vi "Call.vi"(7 "Actor in":refnum<class "Actor.lvclass">, 8 "Error in":errorcluster, 10 "Msg":refnum<class "Msg.lvclass">) -> (0 "Error out":errorcluster, 2 "Msg Output":refnum<class "Msg Output.lvclass">, 5 "Actor out":refnum<class "Actor.lvclass">)   [LabVIEW 2020, in "jettl.lvlib"]
uses:
  jettl.lvlib
  Actor/Actor.lvclass
  Msg Output/Msg Output.lvclass
  Msg/Msg.lvclass
  Default Implementation.vi
  Attributes/Attributes.lvclass
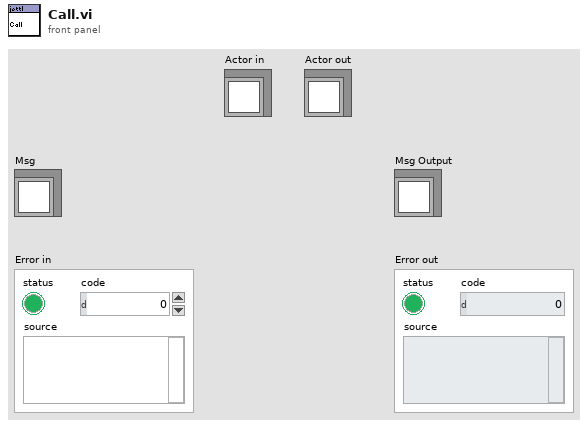
[diagram p1: front panel]
types:
  T1 = typedef "jettl.lvlib/Msgs.ctl" = set{refnum<class "Msg.lvclass">}
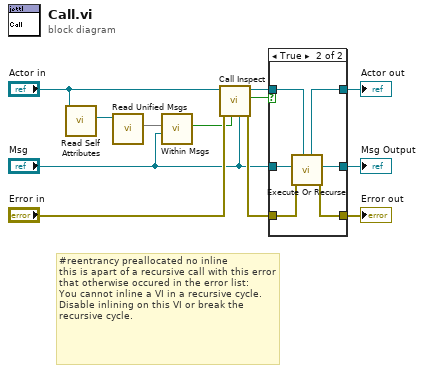
[diagram p0: block diagram]
diagram:
  # "#reentrancy preallocated no inline\nthis is apart of a recursive call with this error that otherwise occured in the error list:\nYou cannot inline a VI in a recursive cycle. Disable inlining on this VI or break the recursive cycle."
  n1 = call-dynamic "Read Self Attributes.vi"("Actor in"="Actor in") -> ("Self Attributes"=w12:refnum<class "Attributes.lvclass">)  [unwired: 10 in]
  n2 = call-dynamic "Read Unified Msgs.vi"("Attributes in"=w12) -> ("Unified Msgs"=w11:T1)  [unwired: 10 in]
  n3 = call "Within Msgs.vi"("Msg"="Msg", "Msgs"=w11) -> ("Within Msgs"=w1:bool)  [unwired: 9 in]
  n4 = call-dynamic "Call Inspect.vi"("Msg"="Msg", "Within Unified Msgs"=w1, "Error in"="Error in", "Actor in"="Actor in") -> ("Error out"=w3:errorcluster, "Proceed"=w5:bool, "Actor out"=w7:refnum<class "Actor.lvclass">)  [unwired: 5 in]
  n5 = case shown="True" w5 {
    tunnel: w7 -> [w14 w20]
    tunnel: [w14 w19] -> w9
    tunnel: "Msg" -> [_ w17]
    tunnel: [w13 w18] -> w8
    tunnel: [_ w16] -> w6
    tunnel: w3 -> [w13 w15]
    frame False {
    }
    frame True {
      n6 = call "Execute Or Recurse.vi"("Actor in"=w20, "Error in"=w15, "Msg"=w17) -> ("Error out"=w18:errorcluster, "Msg Output"=w16:refnum<class "Msg Output.lvclass">, "Actor out"=w19:refnum<class "Actor.lvclass">)  [unwired: 6 in]
    }
  }
  "Actor out" <- w9
  "Error out" <- w8
  "Msg Output" <- w6
